vi "DAQ Calib.vi"(1 "Time Control Parameters":cluster{"# samples":u32, "tiempos (ms)":dbl}, 2 "Calibracion DAQ":T1, 4 "DAQ Device IN":T2) -> (0 "Calibration OUT":dbl[](array[numeric]))   [LabVIEW 2010]
uses:
  <vilib>/measure/NI_MABase.lvlib
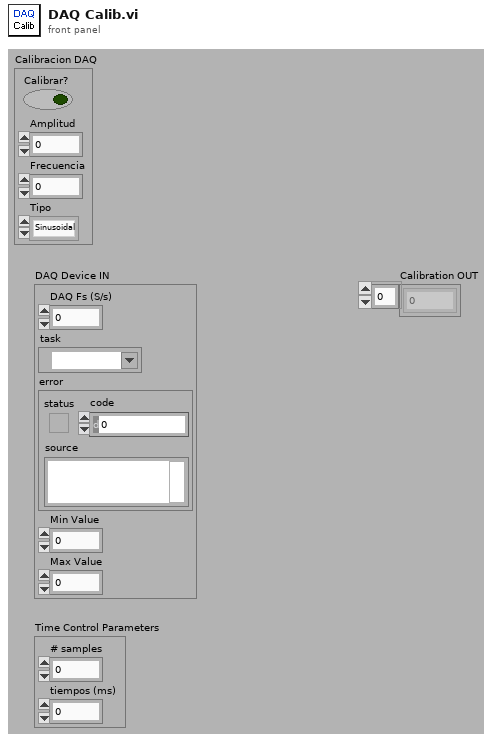
[diagram p1: front panel]
types:
  T1 = cluster{"Calibrar?":bool, "Amplitud":dbl, "Frecuencia":dbl, "Tipo":enum16{"Sinusoidal", "Triangular", "Cuadrada"}}
  T2 = cluster{"DAQ Fs (S/s)":dbl, "task":refnum<k21>, "error":errorcluster, "Min Value":dbl, "Max Value":dbl}
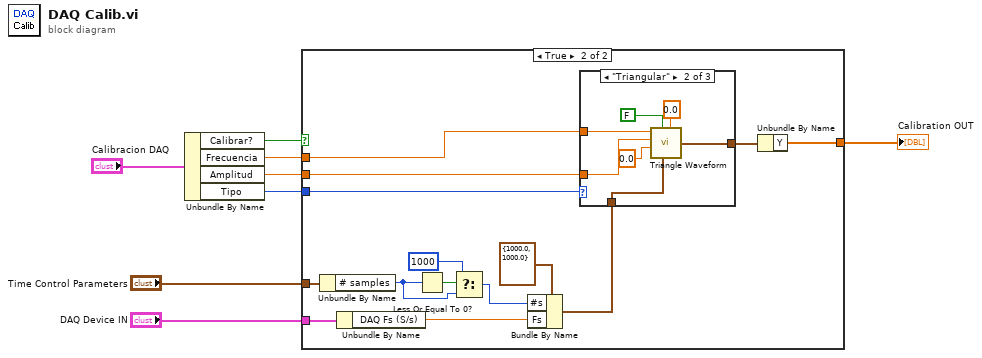
[diagram p0: block diagram]
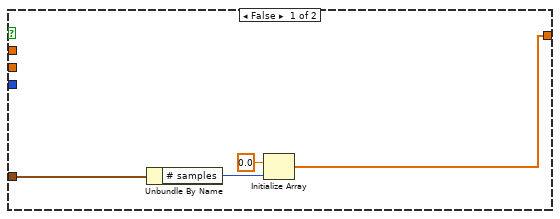
[diagram p2: hidden frame]
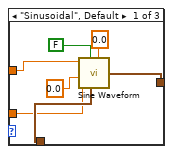
[diagram p3: hidden frame]
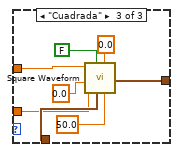
[diagram p4: hidden frame]
diagram:
  n1 = Unbundle By Name("Calibracion DAQ") -> ("Calibrar?"=w4:bool, "Frecuencia"=w5:dbl, "Amplitud"=w6:dbl, "Tipo"=w7:enum16{"Sinusoidal", "Triangular", "Cuadrada"})
  n2 = case shown="True" w4 {
    tunnel: "Time Control Parameters" -> [w10 w21]
    tunnel: "DAQ Device IN" -> [_ w25]
    tunnel: [w9 w20] -> w3
    tunnel: w5 -> [_ w14]
    tunnel: w6 -> [_ w13]
    tunnel: w7 -> [_ w19]
    frame False {
      n3 = Unbundle By Name(w10) -> ("# samples"=w11:u32)
      n4 = Initialize Array(0.0 ("element"), w11) -> (w9:dbl[])
    }
    frame True {
      n5 = Unbundle By Name(w21) -> ("# samples"=w22:u32)
      n6 = Unbundle By Name(w25) -> ("DAQ Fs (S/s)"=w15:dbl)
      n7 = Less Or Equal To 0?(x=w22) -> (x <= 0?=w24:bool)
      n8 = Select(t=u32 1000, s=w24, f=w22) -> (s? t:f=w16:u32)
      n9 = Bundle By Name(cluster=cluster{"Fs":dbl, "#s":dbl} {"Fs"=1000.0, "#s"=1000.0} ("sampling info"), "#s"=w16, "Fs"=w15) -> (w18:cluster{"Fs":dbl, "#s":dbl})
      n10 = case shown="\"Triangular\"" w19 {
        tunnel: w18 -> [w33 w35 w45]
        tunnel: w13 -> [w31 w36 w44]
        tunnel: w14 -> [w30 w37 w43]
        tunnel: [w27 w34 w42] -> w17
        frame "Sinusoidal", Default {
          n11 = call <vilib>:"Sine Waveform.vi"("offset"=0.0, "sampling info"=w33, "reset signal"=FALSE, "phase"=0.0, "amplitude"=w31, "frequency"=w30) -> ("signal out"=w27:waveform(dbl))  [unwired: 4 in, 1 out]
        }
        frame "Triangular" {
          n12 = call <vilib>:"Triangle Waveform.vi"("offset"=0.0, "sampling info"=w35, "reset signal"=FALSE, "phase"=0.0, "amplitude"=w36, "frequency"=w37) -> ("signal out"=w34:waveform(dbl))  [unwired: 4 in, 1 out]
        }
        frame "Cuadrada" {
          n13 = call <vilib>:"Square Waveform.vi"("duty cycle (%)"=50.0, "offset"=0.0, "sampling info"=w45, "reset signal"=FALSE, "phase"=0.0, "amplitude"=w44, "frequency"=w43) -> ("signal out"=w42:waveform(dbl))  [unwired: 3 in, 1 out]
        }
      }
      n14 = Unbundle By Name(w17) -> ("Y"=w20:dbl[])
    }
  }
  "Calibration OUT" <- w3
